vi "Configure Modulation (Frequency).vi"(0 "VISA resource name":refnum<visa-resource-name>, 1 "Enable Frequency Modulation (T:Enable)":bool, 2 "Modulation Frequency (1000.0 Hz)":dbl, 5 "Channel (1: Channel1)":u16(ring) items=["Channel1", "Channel2"], 7 "FM Source (0: Internal)":u16(ring) items=["Internal", "Other Channel", "External"], 9 "Modulation Waveform (0: Sine)":u16(ring) items=["Sine", "Square", "Ramp", "Negative Ramp", "Triangle", "Noise", "Arbitrary Waveform"], 11 "error in (no error)":errorcluster, 12 "Arbitrary Waveform Name (\"ARB1\")":string, 13 "Peak Deviation (1000.0 Hz)":dbl) -> (4 "VISA resource name out":refnum<visa-resource-name>, 15 "error out":errorcluster)   [LabVIEW 2009, in "Agilent 81150.lvlib"]
doc: "Configures and enables frequency modulation (FM). In FM, the frequency of the carrier is varied by the frequency of the modulating waveform. \n\n<B>Note(s):</B>\nThe carrier waveform shape and parameters are set by the Configure Standard Waveform VI."
uses:
  Agilent 81150.lvlib
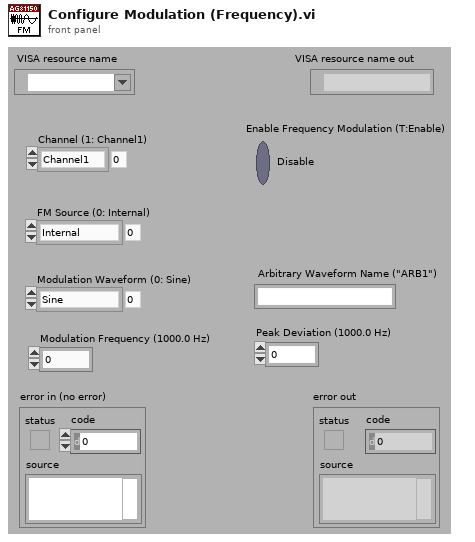
[diagram p1: front panel]
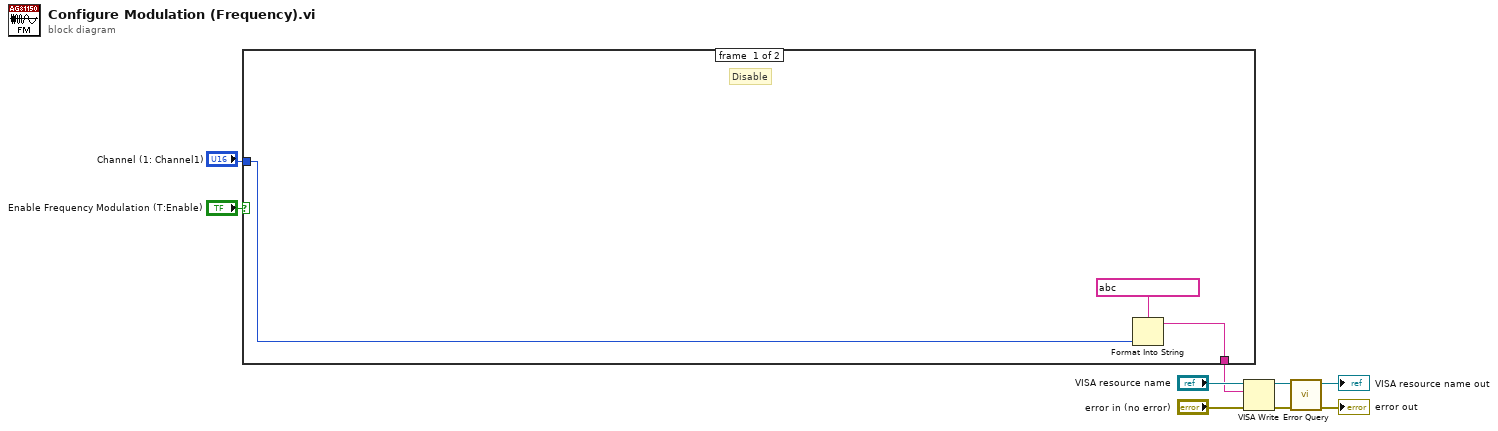
[diagram p0: block diagram]
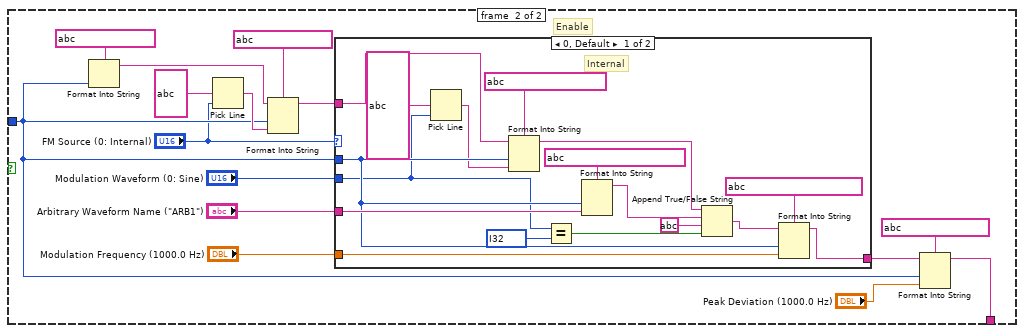
[diagram p2: hidden frame]
diagram:
  n1 = case shown="True" "Enable Frequency Modulation (T:Enable)" {
    tunnel: [w11 w14] -> w3
    tunnel: "Channel (1: Channel1)" -> [w10 w17]
    frame #0 {
      # "Disable"
      n2 = Format Into String(format string=string ?, w10) -> (resulting string=w11:string)  [unwired: 2 in, 1 out]
    }
    frame #1 {
      # "Enable"
      n3 = Format Into String(format string=string ?, w17) -> (resulting string=w13:string)  [unwired: 2 in, 1 out]
      n4 = Pick Line(multi-line string=string ?, line index="FM Source (0: Internal)") -> (output string=w18:string)  [unwired: 1 out]
      n5 = Format Into String(format string=string ?, initial string=w13, w17, w18) -> (resulting string=w20:string)  [unwired: 1 in, 1 out]
      n6 = case shown="0, Default" "FM Source (0: Internal)" {
        tunnel: w17 -> [w38 _]
        tunnel: [w41 w45] -> w26
        tunnel: "Modulation Waveform (0: Sine)" -> [w29 _]
        tunnel: "Modulation Frequency (1000.0 Hz)" -> [w40 _]
        tunnel: "Arbitrary Waveform Name (\"ARB1\")" -> [w39 _]
        tunnel: w20 -> [w30 w45]
        frame #0 {
          w28 = i32 ? items=["Sine", "Square", "Ramp", "Negative Ramp", "Triangle", "Noise", "User"] ("Modulation Waveform (0: Sine)")
          # "Internal"
          n7 = Pick Line(multi-line string=string ?, line index=w29) -> (output string=w36:string)  [unwired: 1 out]
          n8 = Format Into String(format string=string ?, initial string=w30, w38, w36) -> (resulting string=w34:string)  [unwired: 1 in, 1 out]
          n9 = Equal?(x=w29, y=w28) -> (x = y?=w35:bool)
          n10 = Format Into String(format string=string ?, w38, w39) -> (resulting string=w33:string)  [unwired: 2 in, 1 out]
          n11 = Append True/False String(1:w35, 2:string ?, 3:w33, 4:w34) -> (0:w32:string)
          n12 = Format Into String(format string=string ?, initial string=w32, w38, w40) -> (resulting string=w41:string)  [unwired: 1 in, 1 out]
        }
        frame #1 {
          # "Other Channel or External"
        }
      }
      n13 = Format Into String(format string=string ?, initial string=w26, w17, "Peak Deviation (1000.0 Hz)") -> (resulting string=w14:string)  [unwired: 1 in, 1 out]
    }
  }
  n14 = VISA Write(VISA resource name="VISA resource name", write buffer=w3, error in (no error)="error in (no error)") -> (VISA resource name out=w5:refnum<visa-resource-name>, error out=w4:errorcluster)  [unwired: 1 out]
  n15 = call "Error Query.vi"("error in (no error)"=w4, "VISA resource name"=w5) -> ("error out"=→"error out":errorcluster, "VISA resource name out"=→"VISA resource name out":refnum<visa-resource-name>)  [unwired: 8 out]
